vi "Get Thread Interfaces.vi"(11 "Plugin in":refnum<class "Plugin.lvclass">) -> (2 "Plugin Interfaces":refnum<class "Plugin Interface.lvclass">[](array[class]), 3 "Plugin out":refnum<class "Plugin.lvclass">)   [LabVIEW 2021, in "DSF Core.lvlib" / "Plugin.lvclass"]
uses:
  Plugin.lvclass
  Interface/Plugin/Plugin Interface.lvclass
  Plugin.lvclass/Plugin.ctl
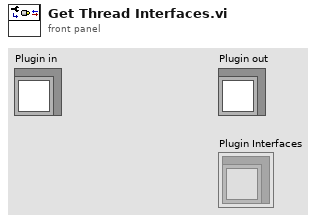
[diagram p1: front panel]
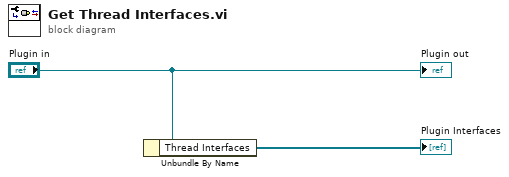
[diagram p0: block diagram]
diagram:
  n1 = Unbundle By Name("Plugin in") -> ("Thread Interfaces"=→"Plugin Interfaces":refnum<class "Plugin Interface.lvclass">[])
  "Plugin out" <- "Plugin in"
